vi "23384_Davis_Poku_Amankwa_Amankwa.DavisPoku.MNE1201.2.1_348253_723087754.vi"() -> ()   [LabVIEW 2018]
panel:
  out "Round Led":bool
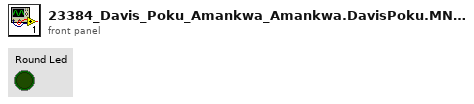
[diagram p1: front panel]
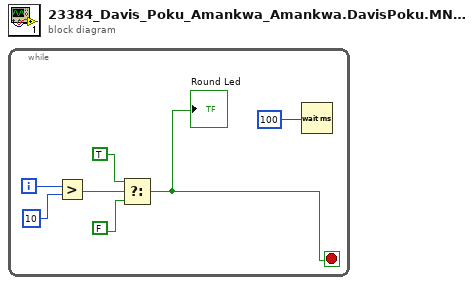
[diagram p0: block diagram]
diagram:
  n1 = while {
    i -> [w3]
    stop <- w2 stop-if-true
    n2 = Greater?(x=w3, y=10) -> (0:w4:bool)
    n3 = Select(t=TRUE, s=w4, f=FALSE) -> (s? t:f=w2:bool)
    "Round Led" <- w2
    n4 = Wait (ms)(milliseconds to wait=100) -> ()  [unwired: 1 out]
  }
